vi "test RTs Only.vi"(8 "error in":errorcluster, 11 "TestCase in":refnum<class "Create Execution Unit.lvclass">) -> (0 "error out":errorcluster, 3 "TestCase out":refnum<class "Create Execution Unit.lvclass">)   [LabVIEW 2023, in "Create Execution Unit.lvclass"]
uses:
  Create Execution Unit.lvclass
  Create Execution Unit.lvclass/Create Execution Unit.ctl
  <vilib>/addons/_JKI Toolkits/VI Tester/TestCase.llb/TestCase.lvclass
  Scripting/Ballard MIL-STD-1553 Scripting.lvlib
  Engine/Implementation/Execution Unit Factory/Execution Unit Factory.lvclass
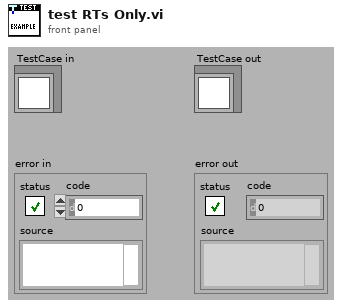
[diagram p1: front panel]
types:
  T1 = cluster{"Hardware File":path, "Parameters File":path}
  T2 = typedef "Custom Device API.lvlib/Custom Device Item Ref.ctl" = u64
  T3 = typedef "Ballard MIL-STD-1553 Engine Support.lvlib/Interfaces.lvlib/Execution Unit Information.ctl" = cluster{"Execution Unit":refnum<class "Execution Unit.lvclass">, "Incoming Channels":T2[], "Outgoing Channels":T2[], "ReadWrite Channels":T2[]}
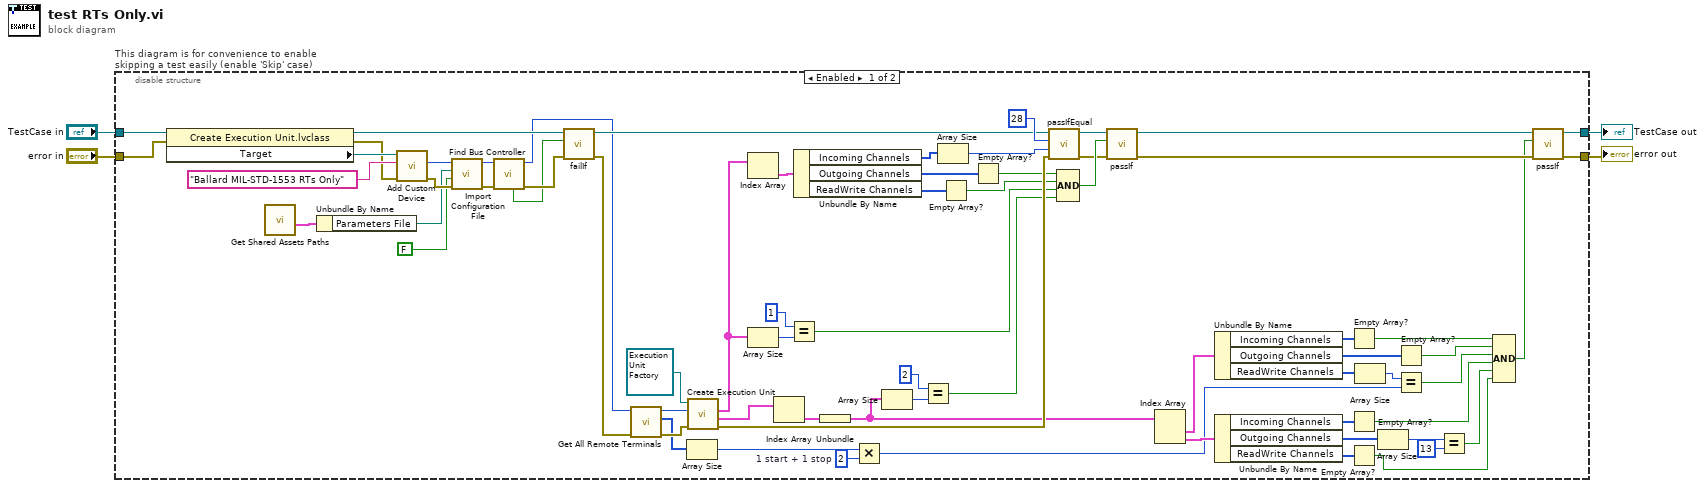
[diagram p0: block diagram]
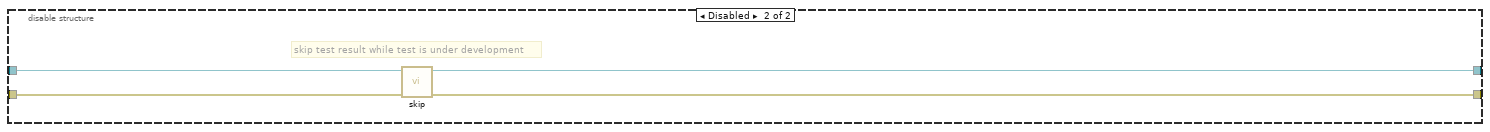
[diagram p2: hidden frame]
diagram:
  n1 = disable-structure "This diagram is for convenience to enable skipping a test easily (enable 'Skip' case)" shown="Enabled" {
    disable-tunnel: "TestCase in" -> [w68 w77]
    disable-tunnel: [w34 w75] -> w1
    disable-tunnel: [w35 w76] -> w3
    disable-tunnel: "error in" -> [w72 w74]
    frame Enabled {
      w38 = 2  # 1 start + 1 stop
      n2 = property class="Create Execution Unit.lvclass"(reference=w68, error in=w72) -> (reference out=w73:refnum<class "Create Execution Unit.lvclass">, error out=w69:errorcluster, "Target"=w70:refnum<k24>)
      n3 = call "Get Shared Assets Paths.vi"() -> ("RTs Only"=w9:T1)  [unwired: 9 in, 2 out]
      n4 = Unbundle By Name(w9) -> ("Parameters File"=w8:path)
      n5 = call "Add Custom Device.vi"("error in"=w69, "name"="Ballard MIL-STD-1553 RTs Only", "target in"=w70) -> ("error out"=w12:errorcluster, "Ballard MIL-STD 1553 custom device"=w13:T2)  [unwired: 6 in, 1 out]
      n6 = call "Import Configuration File.vi"("error in"=w12, "create Tx/Rx folders for subaddresses?"=FALSE, "parameters configuration file path"=w8, "Ballard MIL-STD 1553 custom device in"=w13) -> ("error out"=w10:errorcluster, "Ballard MIL-STD 1553 custom device out"=w11:T2)  [unwired: 6 in]
      n7 = call "Find Bus Controller.vi"("error in"=w10, "port in"=w11) -> ("error out"=w67:errorcluster, "port out"=w44:T2, "found?"=w66:bool)  [unwired: 6 in, 1 out]
      n8 = call-dynamic "failIf.vi"("error in (no error)"=w67, "fail"=w66, "TestCase in"=w73) -> ("error out"=w43:errorcluster, "TestCase out"=w50:refnum<class "Create Execution Unit.lvclass">)  [unwired: 7 in]
      n9 = call "Get All Remote Terminals.vi"("error in"=w43, "port in"=w44) -> ("error out"=w42:errorcluster, "remote terminals"=w40:T2[], "port out"=w41:T2)  [unwired: 7 in]
      n10 = Array Size(array=w40) -> (size(s)=w39:i32)
      n11 = call-dynamic "Create Execution Unit.vi"("error in"=w42, "Item Ref"=w41, "Execution Unit Factory Implementation in"=refnum<class "Execution Unit Factory.lvclass"> refnum) -> ("error out"=w56:errorcluster, "Asynchronous Execution Units"=w48:cluster{"Grouped Execution Units":T3[]}[], "Inline Execution Units"=w49:T3[])  [unwired: 5 in, 1 out]
      n12 = Index Array(array=w49) -> (element=w60:T3)  [unwired: 1 in]
      n13 = Array Size(array=w49) -> (size(s)=w64:i32)
      n14 = Index Array(array=w48) -> (element=w7:cluster{"Grouped Execution Units":T3[]})  [unwired: 1 in]
      n15 = Equal?(x=1, y=w64) -> (x = y?=w52:bool)
      n16 = Unbundle By Name(w60) -> ("Incoming Channels"=w59:T2[], "Outgoing Channels"=w30:T2[], "ReadWrite Channels"=w31:T2[])
      n17 = Unbundle(w7) -> ("Grouped Execution Units"=w6:T3[])
      n18 = Multiply(x=w39, y=w38) -> (x*y=w33:i32)
      n19 = Array Size(array=w6) -> (size(s)=w63:i32)
      n20 = Equal?(x=2, y=w63) -> (x = y?=w51:bool)
      n21 = Array Size(array=w59) -> (size(s)=w55:i32)
      n22 = Empty Array?(array=w31) -> (empty?=w28:bool)
      n23 = Empty Array?(array=w30) -> (empty?=w29:bool)
      n24 = call-dynamic "passIfEqual.vi"("error in (no error)"=w56, "y"=w55, "x"=28 ("size(s)"), "TestCase in"=w50) -> ("error out"=w57:errorcluster, "TestCase out"=w53:refnum<class "Create Execution Unit.lvclass">)  [unwired: 6 in]
      n25 = Compound Arithmetic op=AND(w29, w28, w52, w51) -> (w58:bool)
      n26 = call-dynamic "passIf.vi"("error in (no error)"=w57, "pass"=w58, "TestCase in"=w53) -> ("error out"=w36:errorcluster, "TestCase out"=w37:refnum<class "Create Execution Unit.lvclass">)  [unwired: 7 in]
      n27 = Index Array(array=w6) -> (element #1=w47:T3, element #2=w46:T3)  [unwired: 2 in]
      n28 = Unbundle By Name(w47) -> ("Incoming Channels"=w26:T2[], "Outgoing Channels"=w27:T2[], "ReadWrite Channels"=w45:T2[])
      n29 = Unbundle By Name(w46) -> ("Incoming Channels"=w21:T2[], "Outgoing Channels"=w18:T2[], "ReadWrite Channels"=w20:T2[])
      n30 = Empty Array?(array=w26) -> (empty?=w25:bool)
      n31 = Empty Array?(array=w21) -> (empty?=w19:bool)
      n32 = Empty Array?(array=w20) -> (empty?=w15:bool)
      n33 = Array Size(array=w45) -> (size(s)=w32:i32)
      n34 = Array Size(array=w18) -> (size(s)=w17:i32)
      n35 = Empty Array?(array=w27) -> (empty?=w24:bool)
      n36 = Equal?(x=w32, y=w33) -> (x = y?=w23:bool)
      n37 = Equal?(x=w17, y=13) -> (x = y?=w14:bool)
      n38 = Compound Arithmetic op=AND(w25, w24, w23, w19, w14, w15) -> (w22:bool)
      n39 = call-dynamic "passIf.vi"("error in (no error)"=w36, "pass"=w22, "TestCase in"=w37) -> ("error out"=w35:errorcluster, "TestCase out"=w34:refnum<class "Create Execution Unit.lvclass">)  [unwired: 7 in]
    }
    frame Disabled {
      # "skip test result while test is under development"
      n40 = call <vilib>:"skip.vi"("error in (no error)"=w74, "TestCase in"=w77) -> ("error out"=w76:errorcluster, "TestCase out"=w75:refnum<class "Create Execution Unit.lvclass">)  [unwired: 8 in]
    }
  }
  "error out" <- w3
  "TestCase out" <- w1
